vi "Falling Edge.vi"(11 "signal":bool) -> (3 "falling edge":bool)   [LabVIEW 2017]
doc: "Returns TRUE for one call when signal changes from TRUE to FALSE."
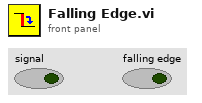
[diagram p1: front panel]
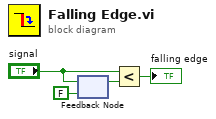
[diagram p0: block diagram]
diagram:
  n1 = feedback #1(FALSE ("signal")) -> (w2:bool)
  n2 = feedback-in #1("signal") -> ()
  n3 = Less?(x="signal", y=w2) -> (x < y?=→"falling edge":bool)
